vi "Autonomous Independent.vi"   [LabVIEW 2012]
doc: "This VI is called when autonomous begins, and will automatically be terminated when autonomous ends. You can carry out timed or sensor driven robot movement independently without needing to return to the caller."
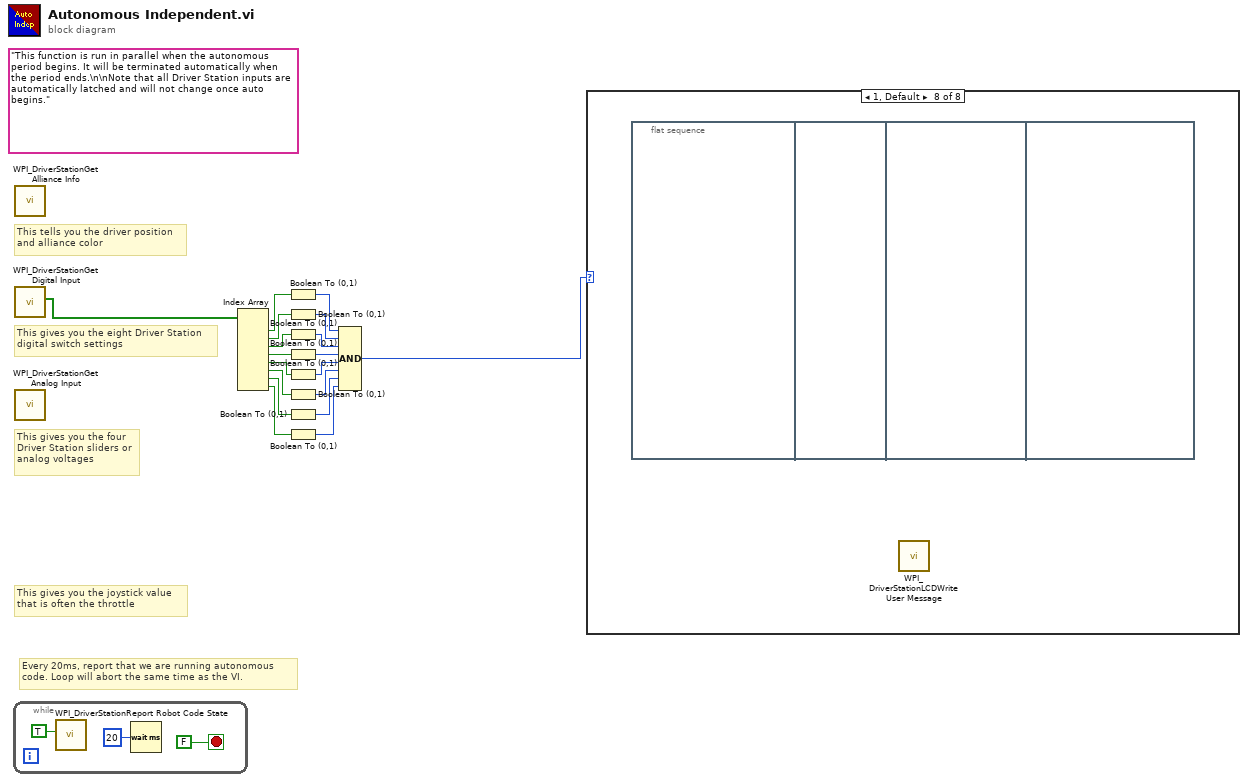
[diagram p0: block diagram]
diagram:
  (unwired) "This function is run in parallel when the autonomous period begins. It will be terminated automatically when the period ends.\n\nNote that all Driver Station inputs are automatically latched and will not change once auto begins."
  # "Every 20ms, report that we are running autonomous\ncode. Loop will abort the same time as the VI."
  # "This gives you the joystick value\nthat is often the throttle"
  # "This tells you the driver position\nand alliance color"
  # "This gives you the eight Driver Station\ndigital switch settings"
  # "This gives you the four\nDriver Station sliders or\nanalog voltages"
  n1 = while {
    stop <- FALSE stop-if-true
    n2 = call <vilib>:"WPI_DriverStationReport Robot Code State.vi"("Autonomous"=TRUE) -> ()  [unwired: 10 in, 1 out]
    n3 = Wait (ms)(milliseconds to wait=u32 20) -> ()  [unwired: 1 out]
  }
  n4 = call <vilib>:"WPI_DriverStationGet Alliance Info.vi"() -> ()  [unwired: 12 out]
  n5 = call <vilib>:"WPI_DriverStationGet Digital Input.vi"() -> ("Driver Station Digital Input (1-8)"=w18:bool[])  [unwired: 11 out]
  n6 = call <vilib>:"WPI_DriverStationGet Analog Input.vi"() -> ()  [unwired: 12 out]
  n7 = Index Array(array=w18) -> (element #1=w16:bool, element #2=w15:bool, element #3=w12:bool, element #4=w8:bool, element #5=w11:bool, element #6=w7:bool, element #7=w3:bool, element #8=w2:bool)  [unwired: 8 in]
  n8 = Boolean To (0,1)(Boolean=w16) -> (0, 1=w17:i16)
  n9 = Boolean To (0,1)(Boolean=w15) -> (0, 1=w14:i16)
  n10 = Boolean To (0,1)(Boolean=w12) -> (0, 1=w13:i16)
  n11 = Boolean To (0,1)(Boolean=w8) -> (0, 1=w9:i16)
  n12 = Boolean To (0,1)(Boolean=w11) -> (0, 1=w10:i16)
  n13 = Boolean To (0,1)(Boolean=w7) -> (0, 1=w6:i16)
  n14 = Boolean To (0,1)(Boolean=w3) -> (0, 1=w5:i16)
  n15 = Boolean To (0,1)(Boolean=w2) -> (0, 1=w4:i16)
  n16 = Compound Arithmetic op=AND(w17, w14, w13, w9, w10, w6, w5, w4) -> (w1:i16)
  n17 = case shown="1, Default" w1 {
    frame 2 {
    }
    frame 3 {
    }
    frame 4 {
    }
    frame 5 {
    }
    frame 6 {
    }
    frame 7 {
    }
    frame 8 {
    }
    frame 1, Default {
      n18 = flat-sequence {
        frame #0 {
        }
        frame #1 {
        }
        frame #2 {
        }
        frame #3 {
        }
      }
      n19 = call <vilib>:"WPI_DriverStationLCDWrite User Message.vi"() -> ()  [unwired: 15 in, 1 out]
    }
  }
